vi "succ_or_not.vi"(10 "x":i32) -> (2 "STATUS":string)   [LabVIEW 2025, in "tcv.lvlib" / "tcv.lvclass"]
uses:
  tcv/tcv.lvclass
  tcv/tcv.lvclass/tcv.ctl
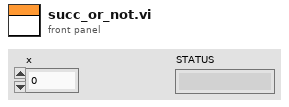
[diagram p1: front panel]
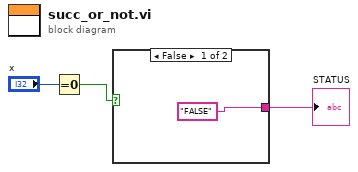
[diagram p0: block diagram]
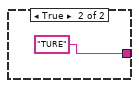
[diagram p2: hidden frame]
diagram:
  n1 = Equal To 0?(x="x") -> (x = 0?=w3:bool)
  n2 = case shown="False" w3 {
    tunnel: ["FALSE" "TURE"] -> w2
    frame False {
    }
    frame True {
    }
  }
  "STATUS" <- w2
